vi "Control_Layer_7-17-15.vi"(8 "stop":bool, 10 "Active Axes":bool[](array[boolean]), 11 "Angles":sgl[](array[numeric])=[0.0, 0.0, 0.0, 0.0, 0.0]) -> ()   [LabVIEW 2014]
uses:
  <vilib>/Platform/TimedLoop/XDataNode/timing_clust.ctl
  <vilib>/Platform/TimedLoop/XDataNode/nitl_modes.ctl
  <vilib>/Platform/TimedLoop/XDataNode/wakeup.ctl
  <vilib>/FPGAPlugInAG/cRIO-9068/niLvFpga_Open_cRIO-9068.vi
  <vilib>/rvi/interface/common/dynamic/niFpgaDynamicAddResources.vi
  <vilib>/Utility/error.llb/Error Cluster From Error Code.vi
  <vilib>/rvi/errors/niLvFpgaAdjustHostInterfaceError.vi
  <vilib>/addons/control/pid/pid.llb/PID (DBL).vi
  <vilib>/FPGAPlugInAG/Dynamic/niLvFpga_Close_Dynamic.vi
  <vilib>/rvi/interface/nirviOpenFPGA/nirviOpenFPGA.xnode
  FPGA Bitfiles/MotorControl_FPGATarget_RobotControl_55TRSUIRMao.lvbitx
  <vilib>/rvi/interface/nirviReadWriteControl/nirviReadWriteControl.xnode
  <vilib>/platform/TimedLoop/XDataNode/XDataNode.xnode
  <vilib>/rvi/interface/nirviCloseFPGA/nirviCloseFPGA.xnode
  <vilib>/rvi/interface/Simulation/niFpgaSimulationCallBeginRW.vi
  NiFpgaLv.dll
  <vilib>/addons/control/pid/NI_PID_pid.lvlib
  <vilib>/Platform/TimedLoop/XDataNode/XDNodeRunTimeDep.lvlib
panel:
  in  "Motor Variables":T1={"Motor 1 Variables"={"Motor 1 P Gains"={"proportional gain (Kc)"=3.0, "integral time (Ti, min)"=0.0, "derivative time (Td, min)"=0.0}, "Motor 1 V Gains"={"proportional gain (Kc)"=0.001, "integral time (Ti, min)"=0.0001, "derivative time (Td, min)"=0.0}, "Velocity Limits"={"output high"=40.0, "output low"=-40.0}, "Duty Cycle Limits"={"output high"=0.6, "output low"=-0.6}}, "Motor 2 Variables"={"Motor 2 P Gains"={"proportional gain (Kc)"=2.0, "integral time (Ti, min)"=0.0, "derivative time (Td, min)"=0.0}, "Motor 2 V Gains"={"proportional gain (Kc)"=0.002, "integral time (Ti, min)"=0.0003, "derivative time (Td, min)"=0.0}, "Velocity Limits"={"output high"=40.0, "output low"=-40.0}, "Duty Cycle Limits"={"output high"=0.6, "output low"=-0.6}}, "Motor 3 Variables"={"Motor 3 P Gains"={"proportional gain (Kc)"=2.0, "integral time (Ti, min)"=0.0, "derivative time (Td, min)"=0.0}, "Motor 3 V Gains"={"proportional gain (Kc)"=0.004, "integral time (Ti, min)"=0.0003, "derivative time (Td, min)"=0.0}, "Velocity Limits"={"output high"=40.0, "output low"=-40.0}, "Duty Cycle Limits"={"output high"=0.6, "output low"=-0.6}}, "Motor 4 Variables"={"Motor 4 P Gains"={"proportional gain (Kc)"=3.0, "integral time (Ti, min)"=0.0, "derivative time (Td, min)"=0.0}, "Motor 4 V Gains"={"proportional gain (Kc)"=0.0004, "integral time (Ti, min)"=0.0001, "derivative time (Td, min)"=0.0}, "Velocity Limits"={"output high"=40.0, "output low"=-40.0}, "Duty Cycle Limits"={"output high"=0.6, "output low"=-0.6}}, "Motor 5 Variables"={"Motor 5 P Gains"={"proportional gain (Kc)"=3.0, "integral time (Ti, min)"=0.0, "derivative time (Td, min)"=0.0}, "Motor 5 V Gains"={"proportional gain (Kc)"=0.0004, "integral time (Ti, min)"=0.0001, "derivative time (Td, min)"=0.0}, "Velocity Limits"={"output high"=40.0, "output low"=-40.0}, "Duty Cycle Limits"={"output high"=0.6, "output low"=-0.6}}}
  out "Motor 5 Velocity":cluster{dbl[], dbl[]}(graph)
  out "Motor 5 Position":cluster{dbl[], dbl[]}(graph)
  out "Motor 4 Velocity":cluster{dbl[], dbl[]}(graph)
  out "Motor 4 Position":cluster{dbl[], dbl[]}(graph)
  out "Motor 3 Velocity":cluster{dbl[], dbl[]}(graph)
  out "Motor 3 Position":cluster{dbl[], dbl[]}(graph)
  out "Motor 2 Velocity":cluster{dbl[], dbl[]}(graph)
  out "Motor 2 Position":cluster{dbl[], dbl[]}(graph)
  out "Motor 1 Velocity":cluster{dbl[], dbl[]}(graph)
  out "Motor 1 Position":cluster{dbl[], dbl[]}(graph)
  out "Colision?":bool
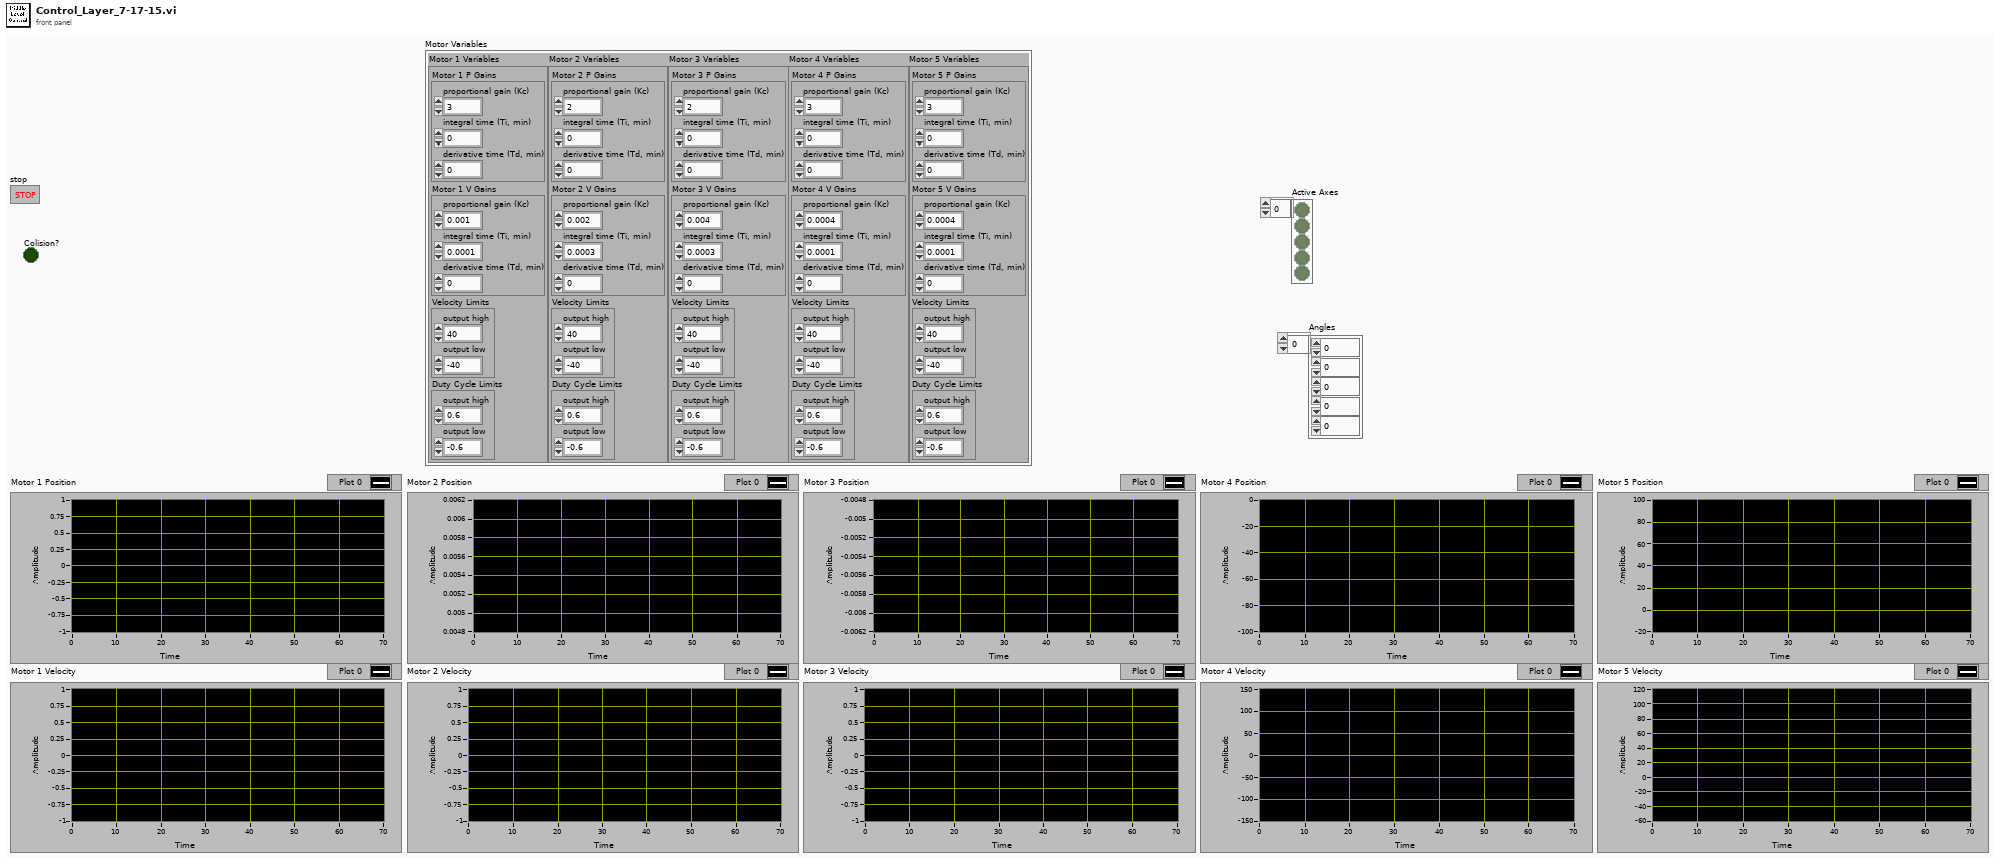
[diagram p1: front panel]
types:
  T1 = cluster{"Motor 1 Variables":cluster{"Motor 1 P Gains":cluster{"proportional gain (Kc)":dbl, "integral time (Ti, min)":dbl, "derivative time (Td, min)":dbl}, "Motor 1 V Gains":cluster{"proportional gain (Kc)":dbl, "integral time (Ti, min)":dbl, "derivative time (Td, min)":dbl}, "Velocity Limits":cluster{"output high":dbl, "output low":dbl}, "Duty Cycle Limits":cluster{"output high":dbl, "output low":dbl}}, "Motor 2 Variables":cluster{"Motor 2 P Gains":cluster{"proportional gain (Kc)":dbl, "integral time (Ti, min)":dbl, "derivative time (Td, min)":dbl}, "Motor 2 V Gains":cluster{"proportional gain (Kc)":dbl, "integral time (Ti, min)":dbl, "derivative time (Td, min)":dbl}, "Velocity Limits":cluster{"output high":dbl, "output low":dbl}, "Duty Cycle Limits":cluster{"output high":dbl, "output low":dbl}}, "Motor 3 Variables":cluster{"Motor 3 P Gains":cluster{"proportional gain (Kc)":dbl, "integral time (Ti, min)":dbl, "derivative time (Td, min)":dbl}, "Motor 3 V Gains":cluster{"proportional gain (Kc)":dbl, "integral time (Ti, min)":dbl, "derivative time (Td, min)":dbl}, "Velocity Limits":cluster{"output high":dbl, "output low":dbl}, "Duty Cycle Limits":cluster{"output high":dbl, "output low":dbl}}, "Motor 4 Variables":cluster{"Motor 4 P Gains":cluster{"proportional gain (Kc)":dbl, "integral time (Ti, min)":dbl, "derivative time (Td, min)":dbl}, "Motor 4 V Gains":cluster{"proportional gain (Kc)":dbl, "integral time (Ti, min)":dbl, "derivative time (Td, min)":dbl}, "Velocity Limits":cluster{"output high":dbl, "output low":dbl}, "Duty Cycle Limits":cluster{"output high":dbl, "output low":dbl}}, "Motor 5 Variables":cluster{"Motor 5 P Gains":cluster{"proportional gain (Kc)":dbl, "integral time (Ti, min)":dbl, "derivative time (Td, min)":dbl}, "Motor 5 V Gains":cluster{"proportional gain (Kc)":dbl, "integral time (Ti, min)":dbl, "derivative time (Td, min)":dbl}, "Velocity Limits":cluster{"output high":dbl, "output low":dbl}, "Duty Cycle Limits":cluster{"output high":dbl, "output low":dbl}}}
  T2 = typedef "XDNodeRunTimeDep.lvlib/timing_clust.ctl" = cluster{"Expected End [f-1]":u64, "Actual End [f-1]":u64, "Finished Late? [f-1]":bool, "Expected End [i-1]":u64, "Actual End [i-1]":u64, "Finished Late? [i-1]":bool, "Expected Start [i]":u64, "Actual Start [i]":u64, "Expected Start [f]":u64, "Actual Start [f]":u64, "Source Name":string, "Structure Name":string, "Period":i64, "Deadline":i64, "Offset":i64, "Start":i64, "Priority":i32, "Timeout":i32, "Mode":T3, "Wakeup Reason":T4, "Error":errorcluster, "Source Type":string, "Secondary Source Type":string, "Global End Time":u64, "Global Start Time":u64, "Frame Duration":u64, "Iteration Duration":u64, "Assigned CPU":i32, "I/O Scan Engine Mode":u32}
  T3 = typedef "XDNodeRunTimeDep.lvlib/nitl_modes.ctl" = enum32{"No Change", "Process missed periods, maintain original phase", "Discard missed periods, maintain original phase", "Process missed periods, ignore original phase", "Discard missed periods, ignore original phase"}
  T4 = typedef "XDNodeRunTimeDep.lvlib/wakeup.ctl" = enum32{"Normal", "Aborted", "Asynchronous wakeup", "Timing source error", "Timed loop error", "Timeout"}
  T5 = cluster{"Motor 1 P Gains":cluster{"proportional gain (Kc)":dbl, "integral time (Ti, min)":dbl, "derivative time (Td, min)":dbl}, "Motor 1 V Gains":cluster{"proportional gain (Kc)":dbl, "integral time (Ti, min)":dbl, "derivative time (Td, min)":dbl}, "Velocity Limits":cluster{"output high":dbl, "output low":dbl}, "Duty Cycle Limits":cluster{"output high":dbl, "output low":dbl}}
  T6 = cluster{"Motor 2 P Gains":cluster{"proportional gain (Kc)":dbl, "integral time (Ti, min)":dbl, "derivative time (Td, min)":dbl}, "Motor 2 V Gains":cluster{"proportional gain (Kc)":dbl, "integral time (Ti, min)":dbl, "derivative time (Td, min)":dbl}, "Velocity Limits":cluster{"output high":dbl, "output low":dbl}, "Duty Cycle Limits":cluster{"output high":dbl, "output low":dbl}}
  T7 = cluster{"Motor 3 P Gains":cluster{"proportional gain (Kc)":dbl, "integral time (Ti, min)":dbl, "derivative time (Td, min)":dbl}, "Motor 3 V Gains":cluster{"proportional gain (Kc)":dbl, "integral time (Ti, min)":dbl, "derivative time (Td, min)":dbl}, "Velocity Limits":cluster{"output high":dbl, "output low":dbl}, "Duty Cycle Limits":cluster{"output high":dbl, "output low":dbl}}
  T8 = cluster{"Motor 4 P Gains":cluster{"proportional gain (Kc)":dbl, "integral time (Ti, min)":dbl, "derivative time (Td, min)":dbl}, "Motor 4 V Gains":cluster{"proportional gain (Kc)":dbl, "integral time (Ti, min)":dbl, "derivative time (Td, min)":dbl}, "Velocity Limits":cluster{"output high":dbl, "output low":dbl}, "Duty Cycle Limits":cluster{"output high":dbl, "output low":dbl}}
  T9 = cluster{"Motor 5 P Gains":cluster{"proportional gain (Kc)":dbl, "integral time (Ti, min)":dbl, "derivative time (Td, min)":dbl}, "Motor 5 V Gains":cluster{"proportional gain (Kc)":dbl, "integral time (Ti, min)":dbl, "derivative time (Td, min)":dbl}, "Velocity Limits":cluster{"output high":dbl, "output low":dbl}, "Duty Cycle Limits":cluster{"output high":dbl, "output low":dbl}}
  T10 = cluster{"proportional gain (Kc)":dbl, "integral time (Ti, min)":dbl, "derivative time (Td, min)":dbl}
  T11 = cluster{"Position (Degrees)":dbl, "Numeric":dbl, "Acceleration":dbl, "Cruise_Velocity":dbl, "Deceleration":dbl, "Time_Accelerate":dbl, "Time_2":dbl, "Time_Total":dbl}
  T12 = cluster{"Acceleration":dbl, "Cruise_Velocity":dbl, "Deceleration":dbl, "Time_Accelerate":dbl, "Time_2":dbl, "Time_Total":dbl}
  T13 = cluster{dbl, "Numeric":dbl, "Acceleration":dbl, "Cruise_Velocity":dbl, "Deceleration":dbl, "Time_Accelerate":dbl, "Time_2":dbl, "Time_Total":dbl}
  T14 = cluster{dbl, dbl, "Acceleration":dbl, "Cruise_Velocity":dbl, "Deceleration":dbl, "Time_Accelerate":dbl, "Time_2":dbl, "Time_Total":dbl}
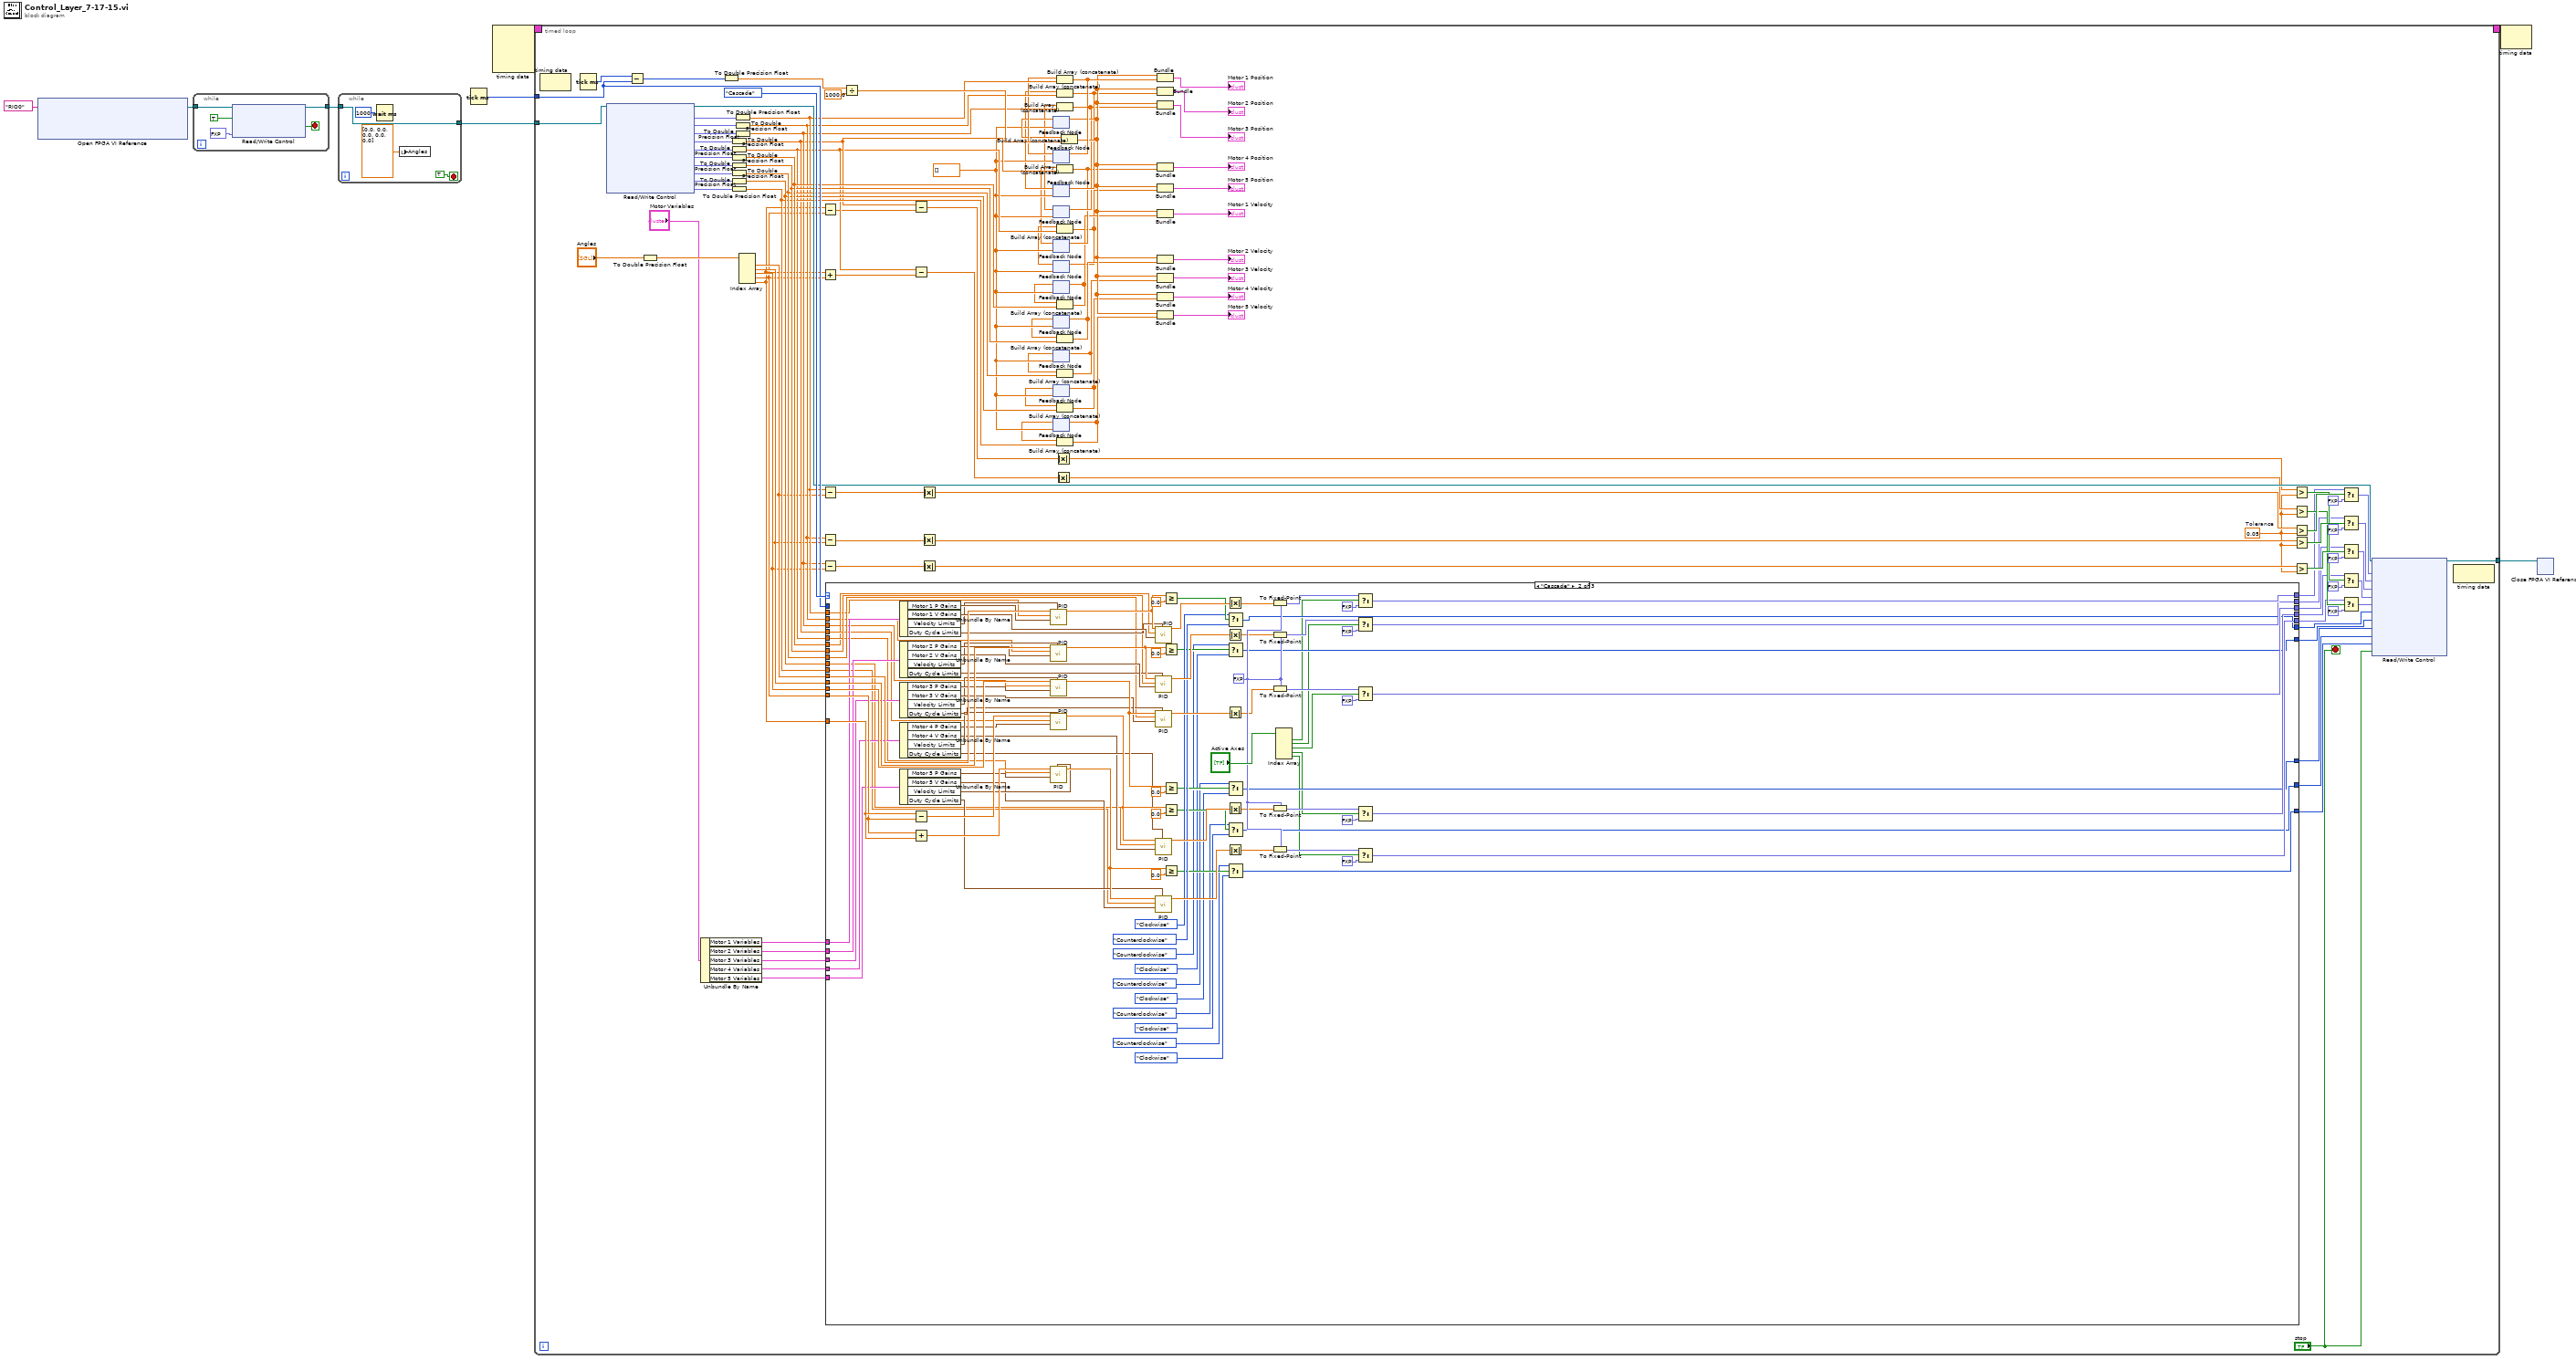
[diagram p0: block diagram]
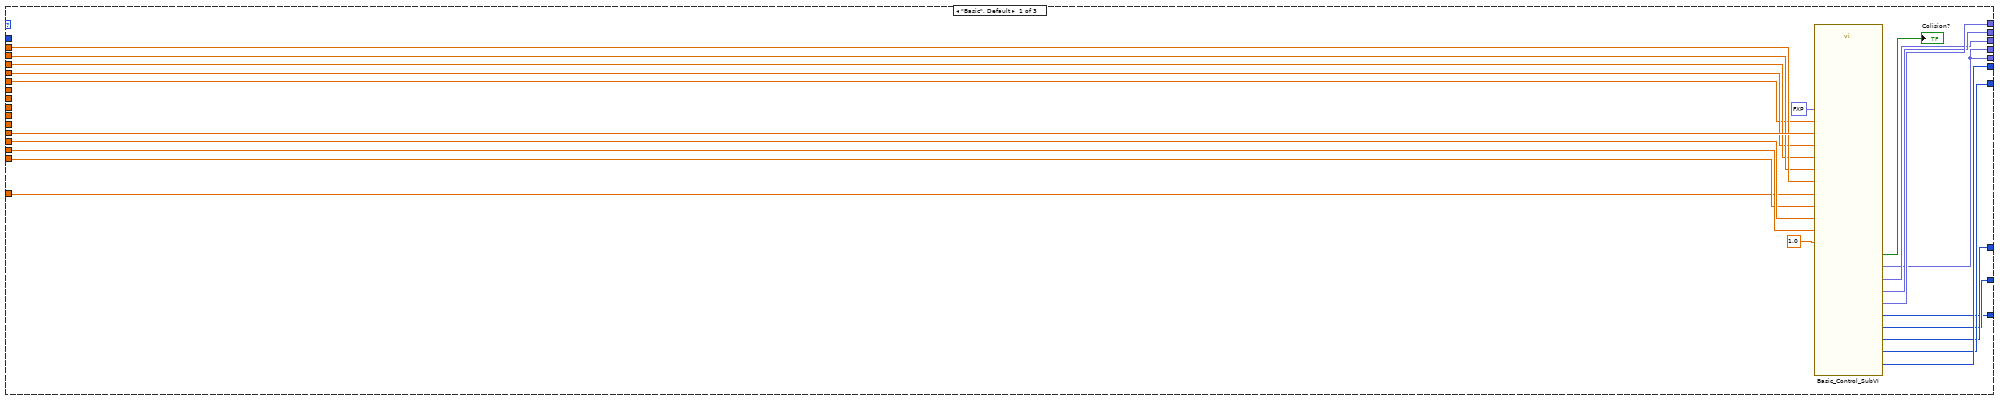
[diagram p2: hidden frame]
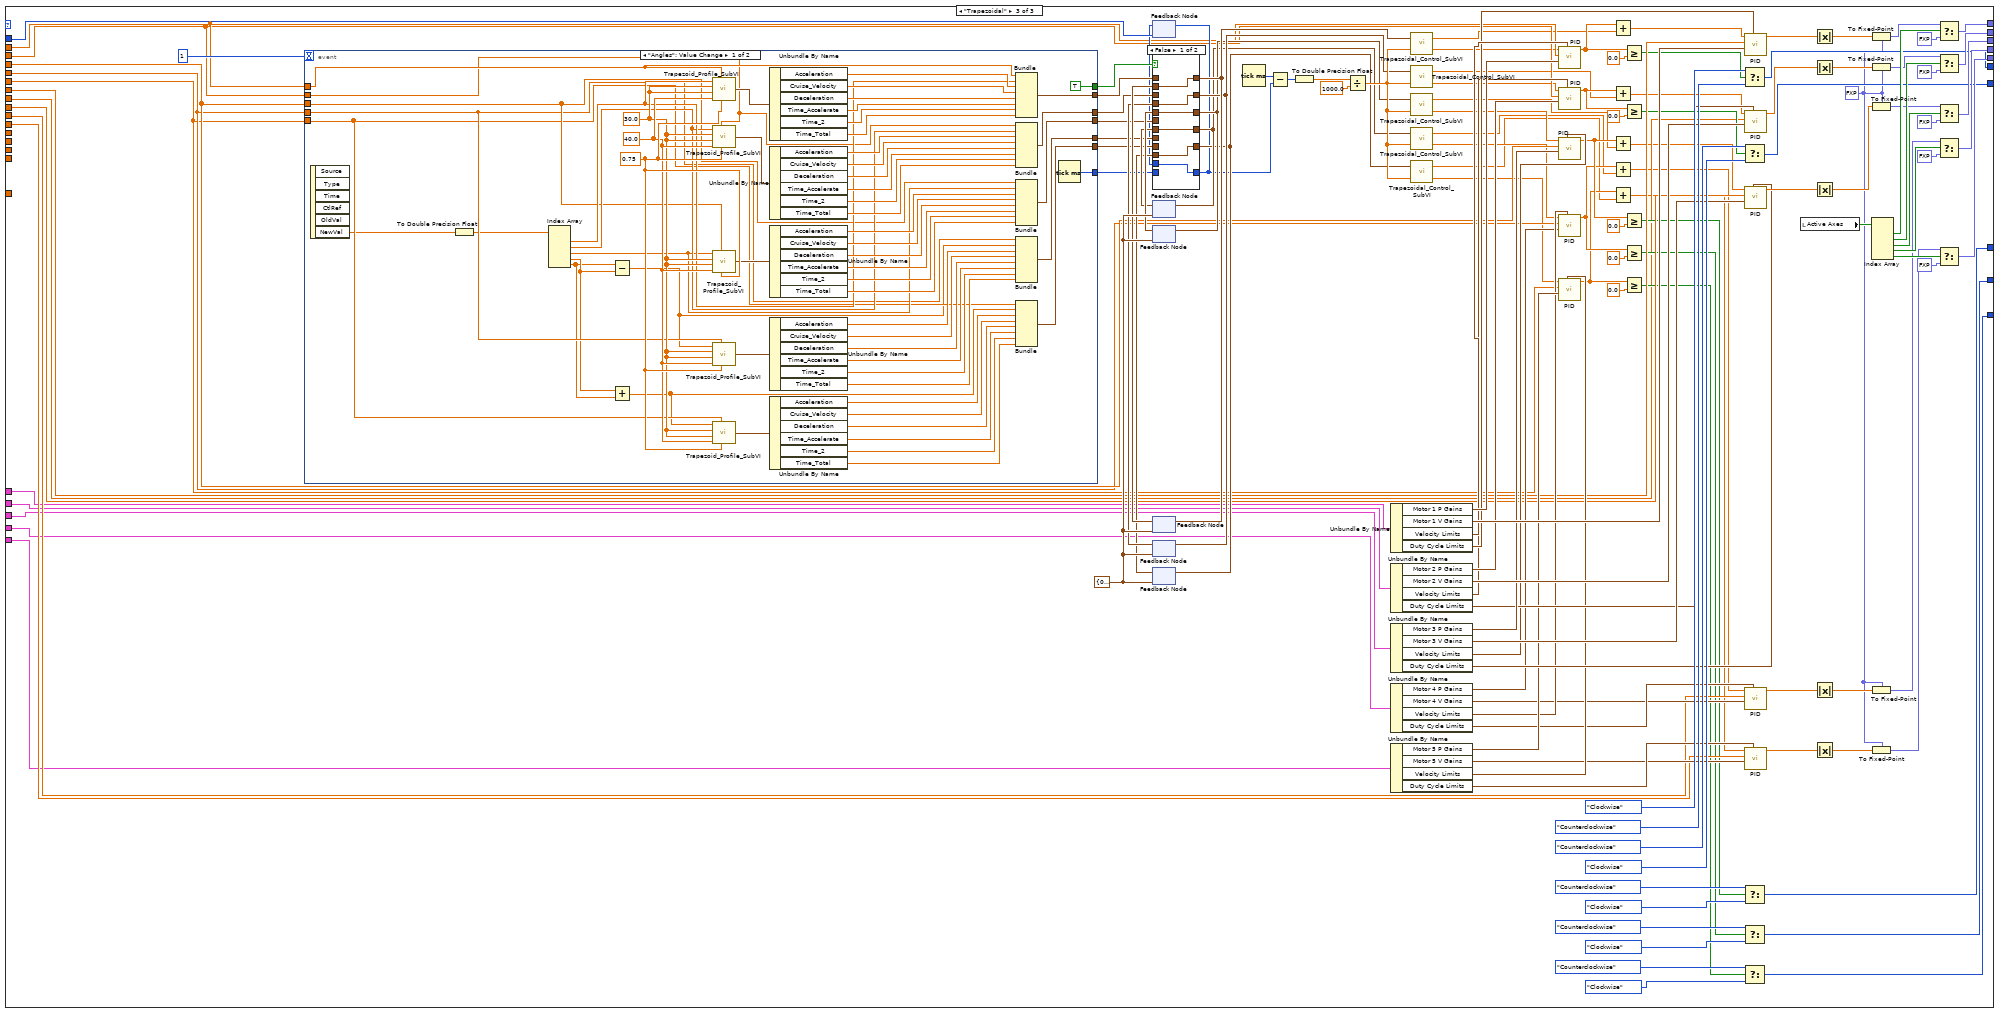
[diagram p3: hidden frame]
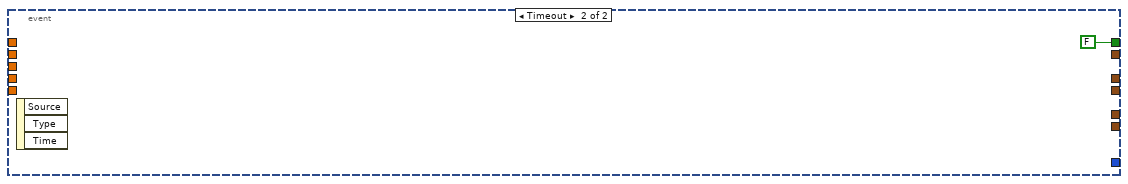
[diagram p5: hidden frame]
diagram:
  n1 = xnode "Open FPGA VI Reference"("resource name"=tag "RIO0") -> ("FPGA VI Reference Out"=w7:refnum<k20>)  [unwired: 1 in, 1 out]
  n2 = while {
    tunnel: w7 -> [w13]
    tunnel: [w10] -> w4
    stop <- w11 stop-if-true
    n3 = xnode "Read/Write Control"("FPGA VI Reference In"=w13, "Go"=TRUE, "Velocity Interval (uSec)"=fxp<+/-,40,24> 5000.0) -> ("FPGA VI Reference Out"=w10:refnum<k20>, "Homed"=w11:bool)  [unwired: 1 in, 1 out]
  }
  n4 = while {
    tunnel: w4 -> [w14]
    tunnel: [w14] -> w3
    stop <- TRUE stop-if-true
    n5 = Wait (ms)(milliseconds to wait=u32 1000) -> ()  [unwired: 1 out]
    n6 = local write "Angles"(sgl[] [0.0, 0.0, 0.0, 0.0, 0.0] ("Angles")) -> ()
  }
  n7 = Tick Count (ms)() -> (millisecond timer value=w5:u32)
  n8 = node-c288() -> (w2:T2)  [unwired: 4 in]
  n9 = timed-loop {
    tunnel: [w132] -> w8
    tunnel: w5 -> [w127]
    tunnel: w3 -> [w129]
    timing: w2 -> [_]
    timing-out: [_] -> w1
    stop <- "stop" stop-if-true
    w49 = dbl[] []
    w70 = 0.05  # Tolerance
    n10 = node-c288() -> ()  [unwired: 1 in, 1 out]
    n11 = Tick Count (ms)() -> (millisecond timer value=w128:u32)
    n12 = xnode "Read/Write Control"("FPGA VI Reference In"=w129) -> ("FPGA VI Reference Out"=w117:refnum<k20>, "Position (Degrees)"=w114:fxp<+/-,40,24>, "Position (Degrees) 2"=w113:fxp<+/-,40,24>, "Position (Degrees) 3"=w112:fxp<+/-,40,24>, "Position (Degrees) 4"=w111:fxp<+/-,40,24>, "Position (Degrees) 5"=w110:fxp<+/-,40,24>, "Velocity (Degrees/Second)"=w109:fxp<+/-,40,24>, "Velocity (Degrees/Second) 2"=w107:fxp<+/-,40,24>, "Velocity (Degrees/Second) 3"=w105:fxp<+/-,40,24>, "Velocity (Degrees/Second) 4"=w103:fxp<+/-,40,24>, "Velocity (Degrees/Second) 5"=w101:fxp<+/-,40,24>)  [unwired: 1 in, 1 out]
    n13 = Subtract(x=w128, y=w127) -> (x-y=w126:u32)
    n14 = To Double Precision Float(number="Angles") -> (double precision float=w115:dbl[])
    n15 = Unbundle By Name("Motor Variables") -> ("Motor 1 Variables"=w98:T5, "Motor 2 Variables"=w97:T6, "Motor 3 Variables"=w96:T7, "Motor 4 Variables"=w95:T8, "Motor 5 Variables"=w94:T9)
    n16 = To Double Precision Float(number=w126) -> (double precision float=w124:dbl)
    n17 = To Double Precision Float(number=w111) -> (double precision float=w75:dbl)
    n18 = To Double Precision Float(number=w110) -> (double precision float=w74:dbl)
    n19 = To Double Precision Float(number=w109) -> (double precision float=w108:dbl)
    n20 = To Double Precision Float(number=w107) -> (double precision float=w106:dbl)
    n21 = To Double Precision Float(number=w105) -> (double precision float=w104:dbl)
    n22 = To Double Precision Float(number=w103) -> (double precision float=w102:dbl)
    n23 = To Double Precision Float(number=w101) -> (double precision float=w100:dbl)
    n24 = To Double Precision Float(number=w114) -> (double precision float=w78:dbl)
    n25 = To Double Precision Float(number=w113) -> (double precision float=w77:dbl)
    n26 = To Double Precision Float(number=w112) -> (double precision float=w76:dbl)
    n27 = Index Array(array=w115) -> (element #1=w73:dbl, element #2=w72:dbl, element #3=w71:dbl, element #4=w19:dbl, element #5=w20:dbl)  [unwired: 5 in]
    n28 = Subtract(x=w20, y=w19) -> (x-y=w21:dbl)
    n29 = Add(x=w20, y=w19) -> (x+y=w18:dbl)
    n30 = Subtract(x=w78, y=w73) -> (x-y=w92:dbl)
    n31 = Subtract(x=w77, y=w72) -> (x-y=w89:dbl)
    n32 = Subtract(x=w76, y=w71) -> (x-y=w86:dbl)
    n33 = case shown="\"Cascade\"" enum16{"Basic", "Cascade", "Trapezoidal"}."Cascade" {
      tunnel: w73 -> [w156 w242 _]
      tunnel: w71 -> [w155 w256 _]
      tunnel: w72 -> [w154 w258 _]
      tunnel: w19 -> [w151 w238 _]
      tunnel: w20 -> [w150 w240 _]
      tunnel: w78 -> [w149 w164 w300]
      tunnel: w108 -> [_ w166 w296]
      tunnel: w77 -> [w148 w165 w282]
      tunnel: w76 -> [w147 w163 w299]
      tunnel: w75 -> [w146 w167 w298]
      tunnel: w74 -> [w145 w168 w297]
      tunnel: w106 -> [_ w169 w281]
      tunnel: w104 -> [_ w170 w295]
      tunnel: w102 -> [_ w157 w294]
      tunnel: w100 -> [_ w171 w293]
      tunnel: w127 -> [_ _ w399]
      tunnel: [w144 w204 w371] -> w64
      tunnel: [w143 w201 w370] -> w62
      tunnel: [w142 w198 w369] -> w60
      tunnel: [w141 w194 w368] -> w58
      tunnel: [w141 w192 w367] -> w56
      tunnel: [w140 w188 w346] -> w122
      tunnel: [w139 w175 w345] -> w121
      tunnel: [w138 w174 w344] -> w120
      tunnel: [w137 w173 w343] -> w119
      tunnel: [w136 w172 w342] -> w118
      tunnel: w98 -> [_ w225 w292]
      tunnel: w97 -> [_ w224 w291]
      tunnel: w96 -> [_ w223 w290]
      tunnel: w95 -> [_ w222 w289]
      tunnel: w94 -> [_ w221 w288]
      frame "Basic", Default {
        n34 = call "Basic_Control_SubVI.vi"("Numeric 2"=w146, "Numeric"=w145, "Numeric 10"=w156, "Numeric 8"=w154, "Numeric 9"=w155, "Numeric 7"=w151, "Numeric 6"=w150, "Numeric 3"=w147, "Tolerance"=1.0, "Numeric 4"=w148, "duty cycle (periods) 5"=fxp<+,32,0> 0.39999999990686774 ("duty cycle (periods)"), "Numeric 5"=w149) -> ("Colision?"=→"Colision?":bool, "duty cycle (periods) 4"=w144:fxp<+,32,0>, "Mod1/Drive Direction 2"=w136:enum8{"Clockwise", "Counterclockwise"}, "Mod1/Drive Direction 6"=w140:enum8{"Clockwise", "Counterclockwise"}, "duty cycle (periods) 3"=w143:fxp<+,32,0>, "Mod1/Drive Direction 5"=w139:enum8{"Clockwise", "Counterclockwise"}, "duty cycle (periods) 2"=w142:fxp<+,32,0>, "Mod1/Drive Direction 4"=w138:enum8{"Clockwise", "Counterclockwise"}, "Mod1/Drive Direction 3"=w137:enum8{"Clockwise", "Counterclockwise"}, "duty cycle (periods)"=w141:fxp<+,32,0>)  [unwired: 6 in]
      }
      frame "Cascade" {
        w237 = fxp<+,32,0> 0.0 ("Duty Cycle 1")
        n35 = Unbundle By Name(w225) -> ("Motor 1 P Gains"=w231:T10, "Motor 1 V Gains"=w230:T10, "Velocity Limits"=w229:cluster{"output high":dbl, "output low":dbl}, "Duty Cycle Limits"=w228:cluster{"output high":dbl, "output low":dbl})
        n36 = Unbundle By Name(w224) -> ("Motor 2 P Gains"=w227:T10, "Motor 2 V Gains"=w226:T10, "Velocity Limits"=w217:cluster{"output high":dbl, "output low":dbl}, "Duty Cycle Limits"=w218:cluster{"output high":dbl, "output low":dbl})
        n37 = Unbundle By Name(w223) -> ("Motor 3 P Gains"=w219:T10, "Motor 3 V Gains"=w220:T10, "Velocity Limits"=w215:cluster{"output high":dbl, "output low":dbl}, "Duty Cycle Limits"=w216:cluster{"output high":dbl, "output low":dbl})
        n38 = Unbundle By Name(w222) -> ("Motor 4 P Gains"=w208:T10, "Motor 4 V Gains"=w207:T10, "Velocity Limits"=w210:cluster{"output high":dbl, "output low":dbl}, "Duty Cycle Limits"=w209:cluster{"output high":dbl, "output low":dbl})
        n39 = Unbundle By Name(w221) -> ("Motor 5 P Gains"=w214:T10, "Motor 5 V Gains"=w211:T10, "Velocity Limits"=w213:cluster{"output high":dbl, "output low":dbl}, "Duty Cycle Limits"=w212:cluster{"output high":dbl, "output low":dbl})
        n40 = Subtract(x=w240, y=w238) -> (x-y=w241:dbl)
        n41 = Add(x=w238, y=w240) -> (x+y=w239:dbl)
        n42 = call-poly <vilib>:"PID.vi"("output range"=w229, "PID gains"=w231, "process variable"=w164, "setpoint"=w242) -> ("output"=w252:dbl)  [unwired: 6 in, 1 out]
        n43 = call-poly <vilib>:"PID.vi"("output range"=w217, "PID gains"=w227, "process variable"=w165, "setpoint"=w258) -> ("output"=w248:dbl)  [unwired: 6 in, 1 out]
        n44 = call-poly <vilib>:"PID.vi"("output range"=w215, "PID gains"=w219, "process variable"=w163, "setpoint"=w256) -> ("output"=w251:dbl)  [unwired: 6 in, 1 out]
        n45 = call-poly <vilib>:"PID.vi"("output range"=w210, "PID gains"=w208, "process variable"=w167, "setpoint"=w241) -> ("output"=w250:dbl)  [unwired: 6 in, 1 out]
        n46 = call-poly <vilib>:"PID.vi"("output range"=w213, "PID gains"=w214, "process variable"=w168, "setpoint"=w239) -> ("output"=w249:dbl)  [unwired: 6 in, 1 out]
        n47 = call-poly <vilib>:"PID.vi"("output range"=w228, "PID gains"=w230, "process variable"=w166, "setpoint"=w252) -> ("output"=w243:dbl)  [unwired: 6 in, 1 out]
        n48 = call-poly <vilib>:"PID.vi"("output range"=w218, "PID gains"=w226, "process variable"=w169, "setpoint"=w248) -> ("output"=w247:dbl)  [unwired: 6 in, 1 out]
        n49 = call-poly <vilib>:"PID.vi"("output range"=w216, "PID gains"=w220, "process variable"=w170, "setpoint"=w251) -> ("output"=w244:dbl)  [unwired: 6 in, 1 out]
        n50 = call-poly <vilib>:"PID.vi"("output range"=w209, "PID gains"=w207, "process variable"=w157, "setpoint"=w250) -> ("output"=w245:dbl)  [unwired: 6 in, 1 out]
        n51 = call-poly <vilib>:"PID.vi"("output range"=w212, "PID gains"=w211, "process variable"=w171, "setpoint"=w249) -> ("output"=w246:dbl)  [unwired: 6 in, 1 out]
        n52 = Greater Or Equal?(x=w252, y=0.0) -> (x >= y?=w191:bool)
        n53 = Greater Or Equal?(x=w248, y=0.0) -> (x >= y?=w187:bool)
        n54 = Greater Or Equal?(x=w251, y=0.0) -> (x >= y?=w186:bool)
        n55 = Greater Or Equal?(x=w250, y=0.0) -> (x >= y?=w185:bool)
        n56 = Greater Or Equal?(x=w249, y=0.0) -> (x >= y?=w184:bool)
        n57 = Absolute Value(x=w243) -> (abs(x)=w236:dbl)
        n58 = Select(t=enum8{"Clockwise", "Counterclockwise"}."Clockwise" ("Mod1/Drive Direction"), s=w191, f=enum8{"Clockwise", "Counterclockwise"}."Counterclockwise" ("Mod1/Drive Direction")) -> (s? t:f=w188:enum8{"Clockwise", "Counterclockwise"})
        n59 = Absolute Value(x=w247) -> (abs(x)=w235:dbl)
        n60 = Select(t=enum8{"Clockwise", "Counterclockwise"}."Counterclockwise" ("Mod1/Drive Direction"), s=w187, f=enum8{"Clockwise", "Counterclockwise"}."Clockwise" ("Mod1/Drive Direction")) -> (s? t:f=w175:enum8{"Clockwise", "Counterclockwise"})
        n61 = Absolute Value(x=w244) -> (abs(x)=w234:dbl)
        n62 = Select(t=enum8{"Clockwise", "Counterclockwise"}."Counterclockwise" ("Mod1/Drive Direction"), s=w186, f=enum8{"Clockwise", "Counterclockwise"}."Clockwise" ("Mod1/Drive Direction")) -> (s? t:f=w174:enum8{"Clockwise", "Counterclockwise"})
        n63 = Absolute Value(x=w245) -> (abs(x)=w232:dbl)
        n64 = Select(t=enum8{"Clockwise", "Counterclockwise"}."Counterclockwise" ("Mod1/Drive Direction"), s=w185, f=enum8{"Clockwise", "Counterclockwise"}."Clockwise" ("Mod1/Drive Direction")) -> (s? t:f=w173:enum8{"Clockwise", "Counterclockwise"})
        n65 = Absolute Value(x=w246) -> (abs(x)=w233:dbl)
        n66 = Select(t=enum8{"Clockwise", "Counterclockwise"}."Counterclockwise" ("Mod1/Drive Direction"), s=w184, f=enum8{"Clockwise", "Counterclockwise"}."Clockwise" ("Mod1/Drive Direction")) -> (s? t:f=w172:enum8{"Clockwise", "Counterclockwise"})
        n67 = To Fixed-Point(fixed-point type=w237, number=w236) -> (fixed-point=w205:fxp<+,32,0>)
        n68 = To Fixed-Point(fixed-point type=w237, number=w235) -> (fixed-point=w202:fxp<+,32,0>)
        n69 = To Fixed-Point(fixed-point type=w237, number=w234) -> (fixed-point=w199:fxp<+,32,0>)
        n70 = To Fixed-Point(fixed-point type=w237, number=w232) -> (fixed-point=w195:fxp<+,32,0>)
        n71 = To Fixed-Point(fixed-point type=w237, number=w233) -> (fixed-point=w193:fxp<+,32,0>)
        n72 = Index Array(array="Active Axes") -> (element #1=w162:bool, element #2=w161:bool, element #3=w160:bool, element #4=w159:bool, element #5=w158:bool)  [unwired: 5 in]
        n73 = Select(t=w205, s=w162, f=fxp<+,32,0> 0.0 ("Duty Cycle 1")) -> (s? t:f=w204:fxp<+,32,0>)
        n74 = Select(t=w202, s=w161, f=fxp<+,32,0> 0.0 ("Duty Cycle 1")) -> (s? t:f=w201:fxp<+,32,0>)
        n75 = Select(t=w199, s=w160, f=fxp<+,32,0> 0.0 ("Duty Cycle 1")) -> (s? t:f=w198:fxp<+,32,0>)
        n76 = Select(t=w195, s=w159, f=fxp<+,32,0> 0.0 ("Duty Cycle 1")) -> (s? t:f=w194:fxp<+,32,0>)
        n77 = Select(t=w193, s=w158, f=fxp<+,32,0> 0.0 ("Duty Cycle 1")) -> (s? t:f=w192:fxp<+,32,0>)
      }
      frame "Trapezoidal" {
        w301 = fxp<+,32,0> 0.0 ("Duty Cycle 1")
        w398 = T11 {"Position (Degrees)"=0.0, "Numeric"=0.0, "Acceleration"=0.0, "Cruise_Velocity"=0.0, "Deceleration"=0.0, "Time_Accelerate"=0.0, "Time_2"=0.0, "Time_Total"=0.0}
        n78 = event shown="[0] \"Angles\": Value Change" {
          selector: _ -> [_ _]
          dyn-events: _ -> [_ _]
          timeout: 1 -> [_ _]
          tunnel: w300 -> [w425 _]
          tunnel: w282 -> [w423 _]
          tunnel: w299 -> [w421 _]
          tunnel: w298 -> [w419 _]
          tunnel: w297 -> [w418 _]
          tunnel: [w460 _] -> w395
          tunnel: [w431 _] -> w390
          tunnel: [w430 _] -> w389
          tunnel: [w429 _] -> w388
          tunnel: [w428 _] -> w387
          tunnel: [TRUE FALSE] -> w397
          tunnel: [w426 _] -> w386
          event "Angles": Value Change {
            w468 = 30.0 ("Acceleration")
            w469 = 40.0 ("Vcruise")
            w470 = 0.75 ("MinFrac_Cruise")
            n79 = event-data() -> ("NewVal"=w417:sgl[])  [unwired: 1 in, 5 out]
            n80 = To Double Precision Float(number=w417) -> (double precision float=w416:dbl[])
            n81 = Index Array(array=w416) -> (element #1=w424:dbl, element #2=w422:dbl, element #3=w420:dbl, element #4=w415:dbl, element #5=w414:dbl)  [unwired: 5 in]
            n82 = Subtract(x=w414, y=w415) -> (x-y=w413:dbl)
            n83 = Add(x=w415, y=w414) -> (x+y=w412:dbl)
            n84 = call "Trapezoid_Profile_SubVI.vi"("MinFrac_Cruise"=w470, "Init_Position"=w425, "Vcruise"=w469, "Deceleration"=w468, "Acceleration"=w468, "Final Position"=w424) -> ("Outputs"=w467:T12)
            n85 = call "Trapezoid_Profile_SubVI.vi"("MinFrac_Cruise"=w470, "Init_Position"=w423, "Vcruise"=w469, "Deceleration"=w468, "Acceleration"=w468, "Final Position"=w422) -> ("Outputs"=w432:T12)
            n86 = call "Trapezoid_Profile_SubVI.vi"("MinFrac_Cruise"=w470, "Init_Position"=w421, "Vcruise"=w469, "Deceleration"=w468, "Acceleration"=w468, "Final Position"=w420) -> ("Outputs"=w433:T12)
            n87 = call "Trapezoid_Profile_SubVI.vi"("MinFrac_Cruise"=w470, "Init_Position"=w419, "Vcruise"=w469, "Deceleration"=w468, "Acceleration"=w468, "Final Position"=w413) -> ("Outputs"=w434:T12)
            n88 = call "Trapezoid_Profile_SubVI.vi"("MinFrac_Cruise"=w470, "Init_Position"=w418, "Vcruise"=w469, "Deceleration"=w468, "Acceleration"=w468, "Final Position"=w412) -> ("Outputs"=w435:T12)
            n89 = Unbundle By Name(w467) -> ("Acceleration"=w461:dbl, "Cruise_Velocity"=w462:dbl, "Deceleration"=w463:dbl, "Time_Accelerate"=w464:dbl, "Time_2"=w465:dbl, "Time_Total"=w466:dbl)
            n90 = Unbundle By Name(w432) -> ("Acceleration"=w459:dbl, "Cruise_Velocity"=w458:dbl, "Deceleration"=w457:dbl, "Time_Accelerate"=w456:dbl, "Time_2"=w455:dbl, "Time_Total"=w454:dbl)
            n91 = Unbundle By Name(w433) -> ("Acceleration"=w448:dbl, "Cruise_Velocity"=w449:dbl, "Deceleration"=w450:dbl, "Time_Accelerate"=w451:dbl, "Time_2"=w452:dbl, "Time_Total"=w453:dbl)
            n92 = Unbundle By Name(w434) -> ("Acceleration"=w447:dbl, "Cruise_Velocity"=w446:dbl, "Deceleration"=w445:dbl, "Time_Accelerate"=w444:dbl, "Time_2"=w443:dbl, "Time_Total"=w442:dbl)
            n93 = Unbundle By Name(w435) -> ("Acceleration"=w436:dbl, "Cruise_Velocity"=w437:dbl, "Deceleration"=w438:dbl, "Time_Accelerate"=w439:dbl, "Time_2"=w440:dbl, "Time_Total"=w441:dbl)
            n94 = Bundle(w425, "Numeric"=w424, "Acceleration"=w461, "Cruise_Velocity"=w462, "Deceleration"=w463, "Time_Accelerate"=w464, "Time_2"=w465, "Time_Total"=w466) -> (w460:T13)  [unwired: 1 in]
            n95 = Bundle(w423, "Numeric"=w422, "Acceleration"=w459, "Cruise_Velocity"=w458, "Deceleration"=w457, "Time_Accelerate"=w456, "Time_2"=w455, "Time_Total"=w454) -> (w431:T13)  [unwired: 1 in]
            n96 = Bundle(w421, "Numeric"=w420, "Acceleration"=w448, "Cruise_Velocity"=w449, "Deceleration"=w450, "Time_Accelerate"=w451, "Time_2"=w452, "Time_Total"=w453) -> (w430:T13)  [unwired: 1 in]
            n97 = Bundle(w419, w413, "Acceleration"=w447, "Cruise_Velocity"=w446, "Deceleration"=w445, "Time_Accelerate"=w444, "Time_2"=w443, "Time_Total"=w442) -> (w429:T14)  [unwired: 1 in]
            n98 = Bundle(w418, w412, "Acceleration"=w436, "Cruise_Velocity"=w437, "Deceleration"=w438, "Time_Accelerate"=w439, "Time_2"=w440, "Time_Total"=w441) -> (w428:T14)  [unwired: 1 in]
            n99 = Tick Count (ms)() -> (millisecond timer value=w426:u32)
          }
          event Timeout {
            n100 = event-data() -> ()  [unwired: 1 in, 3 out]
          }
        }
        n101 = feedback #1(w399) -> (w385:u32)
        n102 = feedback #2(w398) -> (w392:T11)
        n103 = feedback #3(w398) -> (w393:T11)
        n104 = feedback #4(w398) -> (w396:T11)
        n105 = feedback #5(w398) -> (w394:T11)
        n106 = feedback #6(w398) -> (w391:T11)
        n107 = case shown="False" w397 {
          tunnel: w396 -> [w405 _]
          tunnel: [w405 w411] -> w380
          tunnel: w395 -> [_ w411]
          tunnel: [w404 w410] -> w379
          tunnel: [w403 w409] -> w378
          tunnel: [w402 w408] -> w377
          tunnel: [w401 w407] -> w376
          tunnel: w394 -> [w404 _]
          tunnel: w393 -> [w403 _]
          tunnel: w392 -> [w402 _]
          tunnel: w391 -> [w401 _]
          tunnel: w390 -> [_ w410]
          tunnel: w389 -> [_ w409]
          tunnel: w388 -> [_ w408]
          tunnel: w387 -> [_ w407]
          tunnel: w386 -> [_ w406]
          tunnel: w385 -> [w400 _]
          tunnel: [w400 w406] -> w373
          frame False {
          }
          frame True {
          }
        }
        n108 = feedback-in #1(w373) -> ()
        n109 = feedback-in #2(w377) -> ()
        n110 = feedback-in #3(w378) -> ()
        n111 = feedback-in #4(w380) -> ()
        n112 = feedback-in #5(w379) -> ()
        n113 = feedback-in #6(w376) -> ()
        n114 = Tick Count (ms)() -> (millisecond timer value=w374:u32)
        n115 = Subtract(x=w374, y=w373) -> (x-y=w383:u32)
        n116 = To Double Precision Float(number=w383) -> (double precision float=w382:dbl)
        n117 = Divide(x=w382, y=1000.0) -> (x/y=w381:dbl)
        n118 = Unbundle By Name(w292) -> ("Motor 1 P Gains"=w326:T10, "Motor 1 V Gains"=w325:T10, "Velocity Limits"=w324:cluster{"output high":dbl, "output low":dbl}, "Duty Cycle Limits"=w323:cluster{"output high":dbl, "output low":dbl})
        n119 = Unbundle By Name(w291) -> ("Motor 2 P Gains"=w322:T10, "Motor 2 V Gains"=w321:T10, "Velocity Limits"=w317:cluster{"output high":dbl, "output low":dbl}, "Duty Cycle Limits"=w318:cluster{"output high":dbl, "output low":dbl})
        n120 = Unbundle By Name(w290) -> ("Motor 3 P Gains"=w319:T10, "Motor 3 V Gains"=w320:T10, "Velocity Limits"=w315:cluster{"output high":dbl, "output low":dbl}, "Duty Cycle Limits"=w316:cluster{"output high":dbl, "output low":dbl})
        n121 = Unbundle By Name(w289) -> ("Motor 4 P Gains"=w308:T10, "Motor 4 V Gains"=w307:T10, "Velocity Limits"=w310:cluster{"output high":dbl, "output low":dbl}, "Duty Cycle Limits"=w309:cluster{"output high":dbl, "output low":dbl})
        n122 = Unbundle By Name(w288) -> ("Motor 5 P Gains"=w314:T10, "Motor 5 V Gains"=w311:T10, "Velocity Limits"=w313:cluster{"output high":dbl, "output low":dbl}, "Duty Cycle Limits"=w312:cluster{"output high":dbl, "output low":dbl})
        n123 = call "Trapezoidal_Control_SubVI.vi"("Current_Time"=w381, "Inputs"=w380) -> ("pSetProfile"=w280:dbl, "vSetProfile"=w273:dbl)
        n124 = call "Trapezoidal_Control_SubVI.vi"("Current_Time"=w381, "Inputs"=w379) -> ("pSetProfile"=w279:dbl, "vSetProfile"=w267:dbl)
        n125 = call "Trapezoidal_Control_SubVI.vi"("Current_Time"=w381, "Inputs"=w378) -> ("pSetProfile"=w278:dbl, "vSetProfile"=w270:dbl)
        n126 = call "Trapezoidal_Control_SubVI.vi"("Current_Time"=w381, "Inputs"=w377) -> ("pSetProfile"=w277:dbl, "vSetProfile"=w264:dbl)
        n127 = call "Trapezoidal_Control_SubVI.vi"("Current_Time"=w381, "Inputs"=w376) -> ("pSetProfile"=w276:dbl, "vSetProfile"=w261:dbl)
        n128 = call-poly <vilib>:"PID.vi"("output range"=w324, "PID gains"=w326, "process variable"=w300, "setpoint"=w280) -> ("output"=w275:dbl)  [unwired: 6 in, 1 out]
        n129 = call-poly <vilib>:"PID.vi"("output range"=w317, "PID gains"=w322, "process variable"=w282, "setpoint"=w279) -> ("output"=w269:dbl)  [unwired: 6 in, 1 out]
        n130 = call-poly <vilib>:"PID.vi"("output range"=w315, "PID gains"=w319, "process variable"=w299, "setpoint"=w278) -> ("output"=w272:dbl)  [unwired: 6 in, 1 out]
        n131 = call-poly <vilib>:"PID.vi"("output range"=w310, "PID gains"=w308, "process variable"=w298, "setpoint"=w277) -> ("output"=w266:dbl)  [unwired: 6 in, 1 out]
        n132 = call-poly <vilib>:"PID.vi"("output range"=w313, "PID gains"=w314, "process variable"=w297, "setpoint"=w276) -> ("output"=w263:dbl)  [unwired: 6 in, 1 out]
        n133 = Add(x=w275, y=w273) -> (x+y=w274:dbl)
        n134 = Add(x=w269, y=w267) -> (x+y=w268:dbl)
        n135 = Add(x=w272, y=w270) -> (x+y=w271:dbl)
        n136 = Add(x=w266, y=w264) -> (x+y=w265:dbl)
        n137 = Add(x=w263, y=w261) -> (x+y=w262:dbl)
        n138 = Greater Or Equal?(x=w275, y=0.0) -> (x >= y?=w287:bool)
        n139 = Greater Or Equal?(x=w269, y=0.0) -> (x >= y?=w286:bool)
        n140 = Greater Or Equal?(x=w272, y=0.0) -> (x >= y?=w285:bool)
        n141 = Greater Or Equal?(x=w266, y=0.0) -> (x >= y?=w284:bool)
        n142 = Greater Or Equal?(x=w263, y=0.0) -> (x >= y?=w283:bool)
        n143 = Select(t=enum8{"Clockwise", "Counterclockwise"}."Clockwise" ("Mod1/Drive Direction"), s=w287, f=enum8{"Clockwise", "Counterclockwise"}."Counterclockwise" ("Mod1/Drive Direction")) -> (s? t:f=w346:enum8{"Clockwise", "Counterclockwise"})
        n144 = Select(t=enum8{"Clockwise", "Counterclockwise"}."Counterclockwise" ("Mod1/Drive Direction"), s=w286, f=enum8{"Clockwise", "Counterclockwise"}."Clockwise" ("Mod1/Drive Direction")) -> (s? t:f=w345:enum8{"Clockwise", "Counterclockwise"})
        n145 = Select(t=enum8{"Clockwise", "Counterclockwise"}."Counterclockwise" ("Mod1/Drive Direction"), s=w285, f=enum8{"Clockwise", "Counterclockwise"}."Clockwise" ("Mod1/Drive Direction")) -> (s? t:f=w344:enum8{"Clockwise", "Counterclockwise"})
        n146 = Select(t=enum8{"Clockwise", "Counterclockwise"}."Counterclockwise" ("Mod1/Drive Direction"), s=w284, f=enum8{"Clockwise", "Counterclockwise"}."Clockwise" ("Mod1/Drive Direction")) -> (s? t:f=w343:enum8{"Clockwise", "Counterclockwise"})
        n147 = Select(t=enum8{"Clockwise", "Counterclockwise"}."Counterclockwise" ("Mod1/Drive Direction"), s=w283, f=enum8{"Clockwise", "Counterclockwise"}."Clockwise" ("Mod1/Drive Direction")) -> (s? t:f=w342:enum8{"Clockwise", "Counterclockwise"})
        n148 = call-poly <vilib>:"PID.vi"("output range"=w323, "PID gains"=w325, "process variable"=w296, "setpoint"=w274) -> ("output"=w332:dbl)  [unwired: 6 in, 1 out]
        n149 = call-poly <vilib>:"PID.vi"("output range"=w318, "PID gains"=w321, "process variable"=w281, "setpoint"=w268) -> ("output"=w336:dbl)  [unwired: 6 in, 1 out]
        n150 = call-poly <vilib>:"PID.vi"("output range"=w316, "PID gains"=w320, "process variable"=w295, "setpoint"=w271) -> ("output"=w333:dbl)  [unwired: 6 in, 1 out]
        n151 = call-poly <vilib>:"PID.vi"("output range"=w309, "PID gains"=w307, "process variable"=w294, "setpoint"=w265) -> ("output"=w334:dbl)  [unwired: 6 in, 1 out]
        n152 = call-poly <vilib>:"PID.vi"("output range"=w312, "PID gains"=w311, "process variable"=w293, "setpoint"=w262) -> ("output"=w335:dbl)  [unwired: 6 in, 1 out]
        n153 = local read "Active Axes"() -> (w375:bool[])
        n154 = Absolute Value(x=w332) -> (abs(x)=w331:dbl)
        n155 = Absolute Value(x=w336) -> (abs(x)=w330:dbl)
        n156 = Absolute Value(x=w333) -> (abs(x)=w329:dbl)
        n157 = Absolute Value(x=w334) -> (abs(x)=w327:dbl)
        n158 = Absolute Value(x=w335) -> (abs(x)=w328:dbl)
        n159 = To Fixed-Point(fixed-point type=w301, number=w331) -> (fixed-point=w306:fxp<+,32,0>)
        n160 = To Fixed-Point(fixed-point type=w301, number=w330) -> (fixed-point=w305:fxp<+,32,0>)
        n161 = To Fixed-Point(fixed-point type=w301, number=w329) -> (fixed-point=w304:fxp<+,32,0>)
        n162 = To Fixed-Point(fixed-point type=w301, number=w327) -> (fixed-point=w303:fxp<+,32,0>)
        n163 = To Fixed-Point(fixed-point type=w301, number=w328) -> (fixed-point=w302:fxp<+,32,0>)
        n164 = Index Array(array=w375) -> (element #1=w366:bool, element #2=w365:bool, element #3=w364:bool, element #4=w363:bool, element #5=w362:bool)  [unwired: 5 in]
        n165 = Select(t=w306, s=w366, f=fxp<+,32,0> 0.0 ("Duty Cycle 1")) -> (s? t:f=w371:fxp<+,32,0>)
        n166 = Select(t=w305, s=w365, f=fxp<+,32,0> 0.0 ("Duty Cycle 1")) -> (s? t:f=w370:fxp<+,32,0>)
        n167 = Select(t=w304, s=w364, f=fxp<+,32,0> 0.0 ("Duty Cycle 1")) -> (s? t:f=w369:fxp<+,32,0>)
        n168 = Select(t=w303, s=w363, f=fxp<+,32,0> 0.0 ("Duty Cycle 1")) -> (s? t:f=w368:fxp<+,32,0>)
        n169 = Select(t=w302, s=w362, f=fxp<+,32,0> 0.0 ("Duty Cycle 1")) -> (s? t:f=w367:fxp<+,32,0>)
      }
    }
    n170 = Divide(x=w124, y=1000.0) -> (x/y=w123:dbl)
    n171 = Subtract(x=w75, y=w21) -> (x-y=w83:dbl)
    n172 = Subtract(x=w74, y=w18) -> (x-y=w80:dbl)
    n173 = Absolute Value(x=w92) -> (abs(x)=w93:dbl)
    n174 = Absolute Value(x=w89) -> (abs(x)=w88:dbl)
    n175 = Absolute Value(x=w86) -> (abs(x)=w87:dbl)
    n176 = feedback #7(w49) -> (w52:dbl[])
    n177 = feedback #8(w49) -> (w54:dbl[])
    n178 = feedback #9(w49) -> (w48:dbl[])
    n179 = feedback #10(w49) -> (w45:dbl[])
    n180 = feedback #11(w49) -> (w44:dbl[])
    n181 = feedback #12(w49) -> (w43:dbl[])
    n182 = feedback #13(w49) -> (w42:dbl[])
    n183 = feedback #14(w49) -> (w40:dbl[])
    n184 = feedback #15(w49) -> (w39:dbl[])
    n185 = feedback #16(w49) -> (w36:dbl[])
    n186 = feedback #17(w49) -> (w34:dbl[])
    n187 = Absolute Value(x=w83) -> (abs(x)=w82:dbl)
    n188 = Absolute Value(x=w80) -> (abs(x)=w81:dbl)
    n189 = Build Array (concatenate)(w54, w78) -> (w53:dbl[])
    n190 = feedback-in #8(w53) -> ()
    n191 = Build Array (concatenate)(w48, w77) -> (w47:dbl[])
    n192 = feedback-in #9(w47) -> ()
    n193 = Build Array (concatenate)(w45, w76) -> (w46:dbl[])
    n194 = feedback-in #10(w46) -> ()
    n195 = Build Array (concatenate)(w44, w75) -> (w24:dbl[])
    n196 = feedback-in #11(w24) -> ()
    n197 = Build Array (concatenate)(w43, w74) -> (w22:dbl[])
    n198 = feedback-in #12(w22) -> ()
    n199 = Build Array (concatenate)(w42, w108) -> (w23:dbl[])
    n200 = feedback-in #13(w23) -> ()
    n201 = Build Array (concatenate)(w40, w106) -> (w41:dbl[])
    n202 = feedback-in #14(w41) -> ()
    n203 = Build Array (concatenate)(w39, w104) -> (w38:dbl[])
    n204 = feedback-in #15(w38) -> ()
    n205 = Build Array (concatenate)(w36, w102) -> (w37:dbl[])
    n206 = feedback-in #16(w37) -> ()
    n207 = Build Array (concatenate)(w34, w100) -> (w35:dbl[])
    n208 = feedback-in #17(w35) -> ()
    n209 = Build Array (concatenate)(w52, w123) -> (w51:dbl[])
    n210 = feedback-in #7(w51) -> ()
    n211 = Bundle(w51, w53) -> (→"Motor 1 Position":cluster{dbl[], dbl[]})  [unwired: 1 in]
    n212 = Bundle(w51, w47) -> (→"Motor 2 Position":cluster{dbl[], dbl[]})  [unwired: 1 in]
    n213 = Bundle(w51, w46) -> (→"Motor 3 Position":cluster{dbl[], dbl[]})  [unwired: 1 in]
    n214 = Bundle(w51, w24) -> (→"Motor 4 Position":cluster{dbl[], dbl[]})  [unwired: 1 in]
    n215 = Bundle(w51, w22) -> (→"Motor 5 Position":cluster{dbl[], dbl[]})  [unwired: 1 in]
    n216 = Bundle(w51, w23) -> (→"Motor 1 Velocity":cluster{dbl[], dbl[]})  [unwired: 1 in]
    n217 = Bundle(w51, w41) -> (→"Motor 2 Velocity":cluster{dbl[], dbl[]})  [unwired: 1 in]
    n218 = Bundle(w51, w38) -> (→"Motor 3 Velocity":cluster{dbl[], dbl[]})  [unwired: 1 in]
    n219 = Bundle(w51, w37) -> (→"Motor 4 Velocity":cluster{dbl[], dbl[]})  [unwired: 1 in]
    n220 = Bundle(w51, w35) -> (→"Motor 5 Velocity":cluster{dbl[], dbl[]})  [unwired: 1 in]
    n221 = Greater?(x=w82, y=w70) -> (0:w66:bool)
    n222 = Greater?(x=w81, y=w70) -> (0:w65:bool)
    n223 = Greater?(x=w93, y=w70) -> (0:w69:bool)
    n224 = Greater?(x=w88, y=w70) -> (0:w68:bool)
    n225 = Greater?(x=w87, y=w70) -> (0:w67:bool)
    n226 = Select(t=w64, s=w69, f=fxp<+,32,0> 0.0 ("Duty Cycle 1")) -> (s? t:f=w63:fxp<+,32,0>)
    n227 = Select(t=w62, s=w68, f=fxp<+,32,0> 0.0 ("Duty Cycle 1")) -> (s? t:f=w61:fxp<+,32,0>)
    n228 = Select(t=w60, s=w67, f=fxp<+,32,0> 0.0 ("Duty Cycle 1")) -> (s? t:f=w59:fxp<+,32,0>)
    n229 = Select(t=w58, s=w66, f=fxp<+,32,0> 0.0 ("Duty Cycle 1")) -> (s? t:f=w57:fxp<+,32,0>)
    n230 = Select(t=w56, s=w65, f=fxp<+,32,0> 0.0 ("Duty Cycle 1")) -> (s? t:f=w55:fxp<+,32,0>)
    n231 = xnode "Read/Write Control"("FPGA VI Reference In"=w117, "Duty Cycle 1"=w63, "Duty Cycle 2"=w61, "Duty Cycle 3"=w59, "Duty Cycle 4"=w57, "Duty Cycle 5"=w55, "Mod1/Drive Direction"=w122, "Mod1/Drive Direction 2"=w121, "Mod1/Drive Direction 3"=w120, "Mod1/Drive Direction 4"=w119, "Mod1/Drive Direction 5"=w118, "Stop"="stop") -> ("FPGA VI Reference Out"=w132:refnum<k20>)  [unwired: 1 in, 1 out]
    n232 = node-c288() -> ()  [unwired: 1 in, 1 out]
  }
  n233 = node-c288(w1) -> ()  [unwired: 1 out]
  n234 = xnode "Close FPGA VI Reference"("FPGA VI Reference In"=w8) -> ()  [unwired: 1 in, 1 out]
